vi "UART Set Baud Rate.vi"(8 "Error In":errorcluster, 9 "Baud Rate (9600)":u32=9600, 10 "UART Channel (0)":u8, 11 "LINX Resource":T1) -> (0 "Error Out":errorcluster, 2 "Actual Baud":u32, 3 "LINX Resource":T1)   [LabVIEW 2014, in "LMH-LINX.lvlib"]
doc: "Set the specified UART channel's baud rate."
uses:
  LMH-LINX.lvlib
  Private/Type Defs/LINX Ref.ctl
  Private/Type Defs/Platform.ctl
  Private/Type Defs/Interface.ctl
  Private/Device/Type Defs/LINX Device Config.ctl
  Private/Device/Type Defs/TCP Config.ctl
  Private/Device/Type Defs/Channels.ctl
  Private/Type Defs/Peripheral.ctl
  Private/Type Defs/Channel FGV States.ctl
  <vilib>/Instr/_visa.llb/VISA Configure Serial Port (Instr).vi
  Private/myRIO/myRIO.lvlib
  Private/Device/Device.lvlib
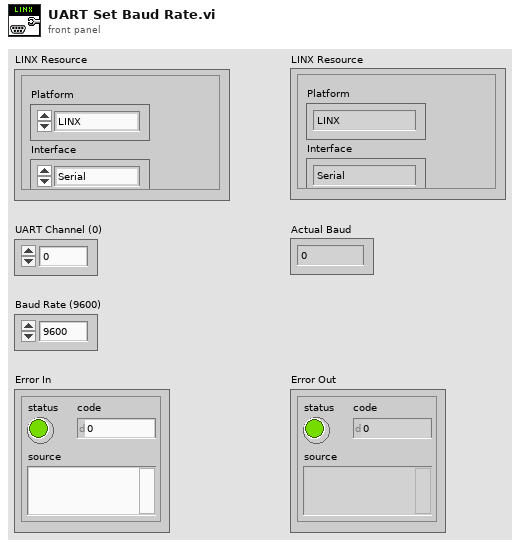
[diagram p1: front panel]
types:
  T1 = typedef "LMH-LINX.lvlib/LINX Ref.ctl" = cluster{"Platform":T2, "Interface":T3, "LINX Device Config":T4}
  T2 = typedef "LMH-LINX.lvlib/Platform.ctl" = enum16{"LINX", "myRIO"}
  T3 = typedef "LMH-LINX.lvlib/Interface.ctl" = enum16{"Serial", "TCP"}
  T4 = typedef "LMH-LINX.lvlib/Device.lvlib/LINX Device Config.ctl" = cluster{"Interface":T3, "COM Port":refnum<visa-resource-name>, "TCP Configuration":T5, "Device Family":u8, "Device ID":u8, "Device Name":string, "TCP Ref":refnum<k5>, "Channels":T6}
  T5 = typedef "LMH-LINX.lvlib/Device.lvlib/TCP Config.ctl" = cluster{"IP Address":string, "Port":u16}
  T6 = typedef "LMH-LINX.lvlib/Channels.ctl" = cluster{"DI":u8[], "DO":u8[], "AI":u8[], "AO":u8[], "PWM":u8[], "QE":u8[], "UART":u8[], "I2C 2":u8[], "SPI":u8[], "CAN":u8[], "Servo":u8[], "AI Ref (V)":dbl, "AO Ref (V)":dbl, "AO Resolution (Bits)":u8}
  T7 = typedef "LMH-LINX.lvlib/Peripheral.ctl" = enum8{"DI", "DO", "AI", "AO", "PWM", "QE", "UART", "I2C", "SPI", "CAN", "Servo"}
  T8 = typedef "LMH-LINX.lvlib/Channel FGV States.ctl" = enum16{"Initialize", "Get", "Set"}
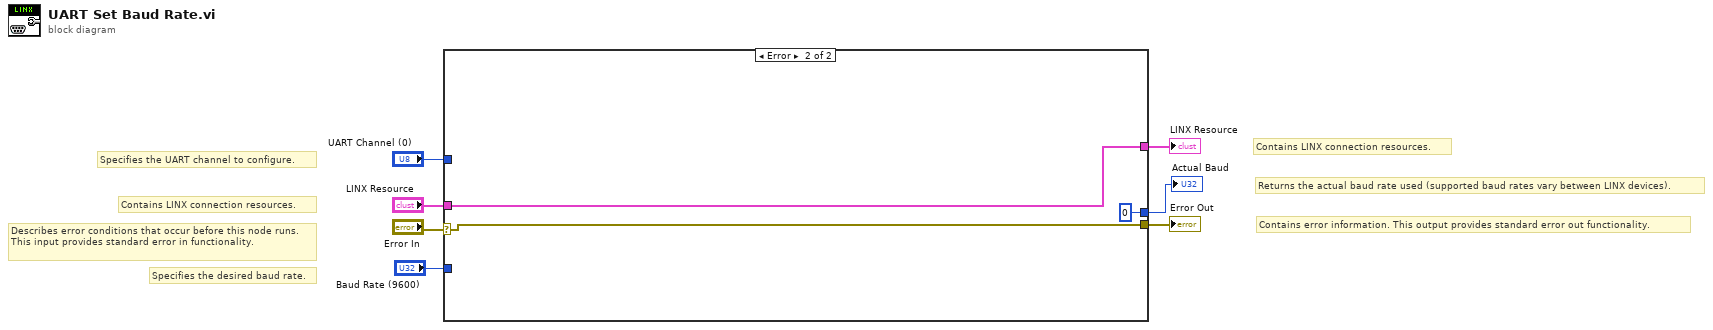
[diagram p0: block diagram]
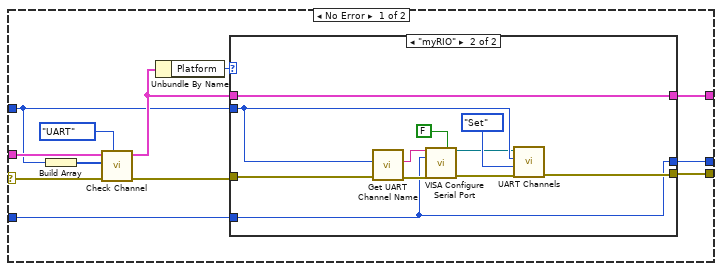
[diagram p2: hidden frame]
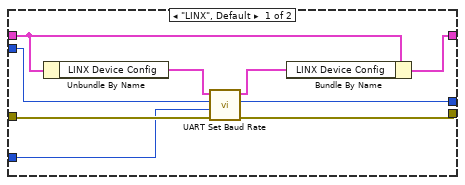
[diagram p3: hidden frame]
diagram:
  # "Returns the actual baud rate used (supported baud rates vary between LINX devices)."
  # "Specifies the desired baud rate."
  # "Specifies the UART channel to configure."
  # "Contains LINX connection resources."
  # "Contains error information. This output provides standard error out functionality."
  # "Contains LINX connection resources."
  # "Describes error conditions that occur before this node runs. This input provides standard error in functionality."
  n1 = case shown="Error" "Error In" {
    selector: "Error In" -> [w9 w42]
    tunnel: [w18 w42] -> w7
    tunnel: [w17 w41] -> w6
    tunnel: "LINX Resource" -> [w16 w41]
    tunnel: "UART Channel (0)" -> [w12 _]
    tunnel: "Baud Rate (9600)" -> [w10 _]
    tunnel: [w8 u32 0 ("Baud Rate (9600)")] -> w1
    frame No Error {
      n2 = Build Array(w12) -> (w13:u8[])
      n3 = call "Check Channel.vi"("Peripheral"=Peripheral."UART", "Error In"=w9, "Channels"=w13, "LINX Resource"=w16) -> ("Error Out"=w14:errorcluster, "LINX Resource"=w15:T1)  [unwired: 5 in, 1 out]
      n4 = Unbundle By Name(w15) -> ("Platform"=w19:T2)
      n5 = case shown="\"myRIO\"" w19 {
        tunnel: w14 -> [w25 w33]
        tunnel: w15 -> [w28 w39]
        tunnel: [w26 w31] -> w18
        tunnel: [w27 w39] -> w17
        tunnel: w12 -> [w22 w35]
        tunnel: w10 -> [w21 w29]
        tunnel: [w20 w29] -> w8
        frame "LINX", Default {
          n6 = Unbundle By Name(w28) -> ("LINX Device Config"=w23:T4)
          n7 = call "UART Set Baud Rate.vi"("Error In"=w25, "Baud Rate (9600)"=w21, "UART Channel"=w22, "LINX Device Config"=w23) -> ("Error Out"=w26:errorcluster, "Actual Baud"=w20:u32, "LINX Device Config"=w24:T4)  [unwired: 5 in]
          n8 = Bundle By Name(cluster=w28, "LINX Device Config"=w24) -> (w27:T1)
        }
        frame "myRIO" {
          n9 = call "Get UART Channel Name.vi"("Error In"=w33, "UART Channel"=w35) -> ("Error Out"=w37:errorcluster, "UART Channel"=w36:string)  [unwired: 8 in]
          n10 = call-poly "VISA Configure Serial Port"("VISA resource name"=w36, "Enable Termination\nChar (T)"=FALSE ("Enable Termination\nChar (T)"), "baud rate (9600)"=w29, "error in (no error)"=w37) -> ("VISA resource name out"=w30:refnum<visa-resource-name>, "error out"=w32:errorcluster)  [unwired: 10 in]
          n11 = call "UART Channels.vi"("Error In"=w32, "Channel State"=Channel_FGV_States."Set", "Channel Number"=w35, "UART Channel"=w30) -> ("Error Out"=w31:errorcluster)  [unwired: 6 in, 1 out]
        }
      }
    }
    frame Error {
    }
  }
  "Error Out" <- w7
  "LINX Resource" <- w6
  "Actual Baud" <- w1
